vi "wmf_get_property.vi"(8 "error in (no error)":errorcluster, 10 "property name":string, 11 "Camera":T1) -> (0 "error out":errorcluster, 1 "Value":sgl, 3 "Camera out":T1, 5 "Auto":bool=TRUE)   [LabVIEW 2024, in "Vision.lvlib"]
uses:
  Vision.lvlib
  camera.ctl
  camera driver.ctl
  bin/LVWMF.dll
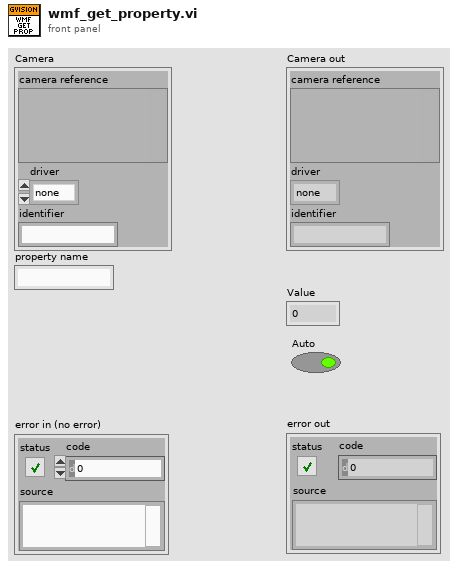
[diagram p1: front panel]
types:
  T1 = typedef "Vision.lvlib/camera.ctl" = cluster{"camera reference":variant, "driver":T2, "identifier":string}
  T2 = typedef "Vision.lvlib/camera driver.ctl" = enum16{"none", "wmf", "imaqdx", "peak"}
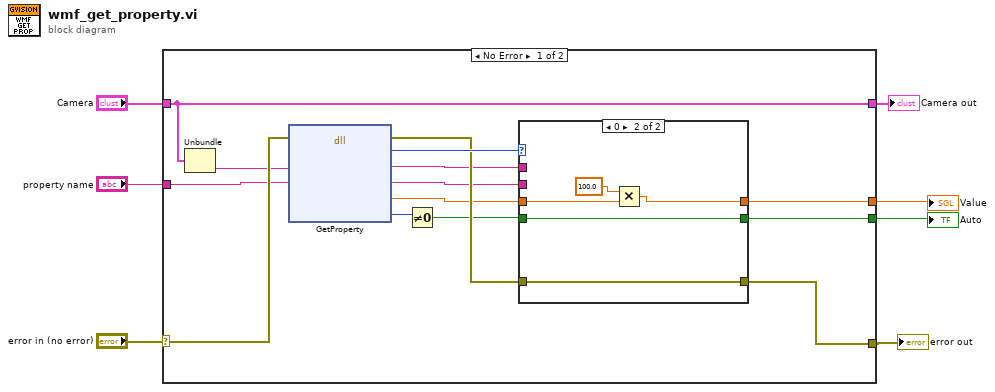
[diagram p0: block diagram]
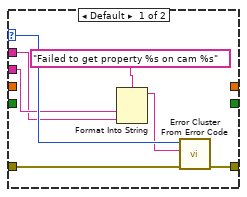
[diagram p2: hidden frame]
diagram:
  n1 = case shown="No Error" "error in (no error)" {
    selector: "error in (no error)" -> [w18 w35]
    tunnel: [w19 w35] -> w6
    tunnel: "property name" -> [w17 _]
    tunnel: [w13 _] -> w4
    tunnel: [w12 _] -> w3
    tunnel: "Camera" -> [w8 w34]
    tunnel: [w8 w34] -> w1
    frame No Error {
      n2 = Unbundle(w8) -> ("identifier"=w9:string)  [unwired: 2 out]
      n3 = dll-call lib="C:/Users/cfang/Desktop/nebraska-silicon-lab/pixel-gantry-control/Gantry/Shared Components/bin/LVWMF.dll" fn="GetProperty"(error in=w18, "camera_name"=w9, "prop name"=w17) -> (error out=w20:errorcluster, "return type"=w21:i32, "camera_name"=w16:string, "prop name"=w15:string, "val"=w14:sgl, "auto"=w11:i32)  [unwired: 4 in, 1 out]
      n4 = Not Equal To 0?(x=w11) -> (x != 0?=w10:bool)
      n5 = case shown="0" w21 {
        selector: w21 -> [w26 _]
        tunnel: w20 -> [w28 w33]
        tunnel: [w27 w33] -> w19
        tunnel: w16 -> [w22 _]
        tunnel: w15 -> [w23 _]
        tunnel: w14 -> [_ w31]
        tunnel: [_ w29] -> w13
        tunnel: w10 -> [_ w32]
        tunnel: [_ w32] -> w12
        frame Default {
          n6 = Format Into String(format string="Failed to get property %s on cam %s" ("error message (\"\")"), w23, w22) -> (resulting string=w24:string)  [unwired: 2 in, 1 out]
          n7 = call <vilib>:"Error Cluster From Error Code.vi"("error in (no error)"=w28, "error message (\"\")"=w24, "error code (0)"=w26) -> ("error out"=w27:errorcluster)  [unwired: 6 in]
        }
        frame 0 {
          n8 = Multiply(x=sgl 100.0, y=w31) -> (x*y=w29:sgl)
        }
      }
    }
    frame Error {
    }
  }
  "error out" <- w6
  "Value" <- w4
  "Auto" <- w3
  "Camera out" <- w1
